vi "GraphSetting Set AllParam (Wave2).vi"(8 "error in (no error)":errorcluster caption="エラー入力（エラーなし）", 10 "Chartグラフパラメータ":T1 {"プロット[]"."Yスケール" items=["振幅1234", "振幅 2", "振幅 33"]; "プロット[]"."Xスケール" items=["XX"]; "プロット[]"."プロット補間" max=5 step=1; "プロット[]"."ポイントスタイル" max=16 step=1; "プロット[]"."太さ" max=5 step=1; "プロット[]"."ラインスタイル" max=4 step=1}, 11 "波形グラフ(Wave)ref(in)":refnum<vi>) -> (0 "error out":errorcluster caption="エラー出力")   [LabVIEW 2014]
uses:
  TypeDef/GraphSetting All.ctl
  TypeDef/GraphSetting Appearance.ctl
  GraphSetting Scale.ctl
  TypeDef/GraphSetting DisplayFormatType.ctl
  TypeDef/GraphSetting Plot.ctl
  TypeDef/GraphSetting Command.ctl
panel:
  # "スケールのスタイルとカラー"
  # "スケール係数"
  # "スケールのスタイルとカラー"
  # "スケールのスタイルとカラー"
  # "スケール係数"
  # "スケールのスタイルとカラー"
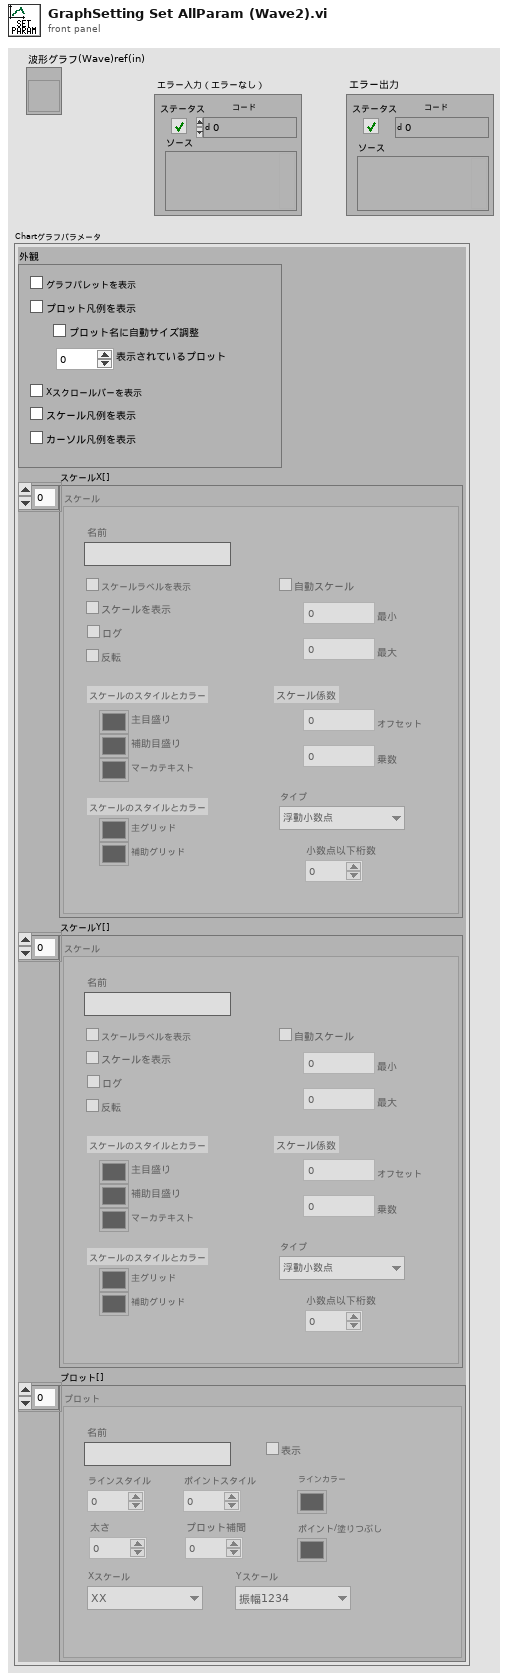
[diagram p1: front panel]
types:
  T1 = typedef "GraphSetting All.ctl" = cluster{"外観":T2, "スケールX[]":T3[], "スケールY[]":T3[], "プロット[]":T5[]}
  T2 = typedef "GraphSetting Appearance.ctl" = cluster{"グラフパレットを表示":bool, "プロット凡例を表示":bool, "プロット名に自動サイズ調整":bool, "表示されているプロット":u32, "Xスクロールバーを表示":bool, "スケール凡例を表示":bool, "カーソル凡例を表示":bool}
  T3 = typedef "GraphSetting Scale.ctl" = cluster{"名前":string, "スケールラベルを表示":bool, "スケールを表示":bool, "ログ":bool, "反転":bool, "自動スケール":bool, "最小":dbl, "最大":dbl, "オフセット":dbl, "乗数":dbl, "主目盛り":u32, "補助目盛り":u32, "マーカテキスト":u32, "主グリッド":u32, "補助グリッド":u32, "タイプ":T4, "小数点以下桁数":u8}
  T4 = typedef "GraphSetting DisplayFormatType.ctl" = enum8{"浮動小数点", "科学", "工学", "バイナリ", "８進数", "１６進数", "相対時間", "時間と日時", "SI"}
  T5 = typedef "GraphSetting Plot.ctl" = cluster{"名前":string, "表示":bool, "ラインスタイル":u8, "太さ":u8, "ポイントスタイル":u8, "プロット補間":u8, "ラインカラー":u32, "ポイント/塗りつぶし":u32, "Xスケール":u16, "Yスケール":u16}
  T6 = typedef "GraphSetting Command.ctl" = enum16{"Get(ref->ctl)", "Set(ctl->ref)"}
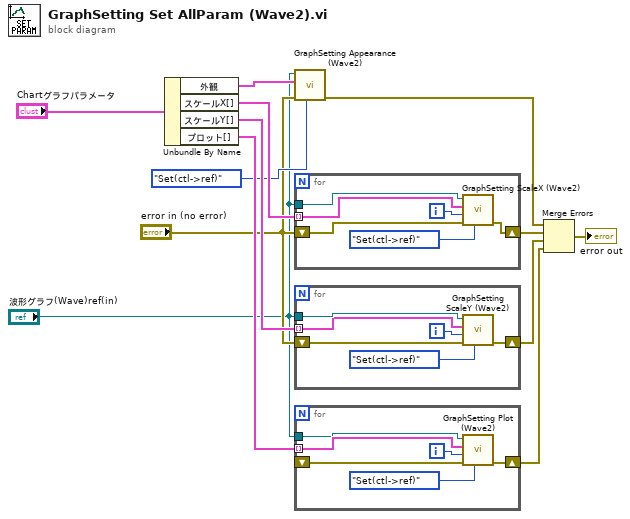
[diagram p0: block diagram]
diagram:
  n1 = Unbundle By Name("Chartグラフパラメータ") -> ("外観"=w9:T2, "スケールX[]"=w13:T3[], "スケールY[]"=w12:T3[], "プロット[]"=w10:T5[])
  n2 = call "GraphSetting Appearance (Wave2).vi"("コマンド"=GraphSetting_Command."Set(ctl->ref)", "error in (no error)"="error in (no error)", "外観(in)"=w9, "波形グラフ(Wave)ref(in)"="波形グラフ(Wave)ref(in)") -> ("error out"=w6:errorcluster)  [unwired: 6 in, 1 out]
  n3 = for {
    tunnel: w13 -> [w19] mode=indexing
    tunnel: "波形グラフ(Wave)ref(in)" -> [w17]
    shift-right: [w15] -> w5
    shift-left: "error in (no error)" -> [w14]
    i -> [w18]
    n4 = call "GraphSetting ScaleX (Wave2).vi"("コマンド"=GraphSetting_Command."Set(ctl->ref)", "error in (no error)"=w14, "アクティブスケール(X)"=w18, "スケール(in)"=w19, "波形グラフ(Wave)ref(in)"=w17) -> ("error out"=w15:errorcluster)  [unwired: 5 in, 1 out]
  }
  n5 = for {
    tunnel: w12 -> [w20] mode=indexing
    shift-right: [w23] -> w4
    shift-left: "error in (no error)" -> [w24]
    tunnel: "波形グラフ(Wave)ref(in)" -> [w25]
    i -> [w22]
    n6 = call "GraphSetting ScaleY (Wave2).vi"("コマンド"=GraphSetting_Command."Set(ctl->ref)", "error in (no error)"=w24, "アクティブスケールY"=w22, "スケール(in)"=w20, "波形グラフ(Wave)ref(in)"=w25) -> ("error out"=w23:errorcluster)  [unwired: 5 in, 1 out]
  }
  n7 = for {
    tunnel: w10 -> [w27] mode=indexing
    shift-right: [w31] -> w3
    shift-left: _ -> [w30]
    tunnel: "波形グラフ(Wave)ref(in)" -> [w26]
    i -> [w29]
    n8 = call "GraphSetting Plot (Wave2).vi"("コマンド"=GraphSetting_Command."Set(ctl->ref)", "error in (no error)"=w30, "アクティブプロット"=w29, "プロット(in)"=w27, "波形グラフ(Wave)ref(in)"=w26) -> ("error out"=w31:errorcluster)  [unwired: 5 in, 1 out]
  }
  n9 = Merge Errors(w6, w5, w4, w3) -> (→"error out":errorcluster)
